vi "StDev Filter Demonstrator.vi"() -> ()   [LabVIEW 2011]
uses:
  <vilib>/ptbypt/NI_PtbyPt.lvlib
  <vilib>/Utility/file.llb/Read From Spreadsheet File (DBL).vi
panel:
  out "Numeric":i32
  out "element":dbl
  in  "shot":dbl=0.8 step=0.01
  out "Waveform Chart":cluster{dbl, dbl}(graph)
  in  "sample":i32=3
  out "Filtered Value":dbl
  in  "StDev":dbl=0.05 step=0.001
  out "StDev":dbl format="%0.2f"
  out "I+N":dbl
  in  "Input":dbl step=0.1
  in  "Manual":bool
  in  "noise":dbl(knob)=0.05940857995844632 scale=0.0..0.1
  in  "Use Time ?":bool=TRUE
  in  "frequency":dbl=0.0001 format="%0.4e"
  in  "amplitude":dbl=0.9999999999999999 step=0.1 format="%0.2f"
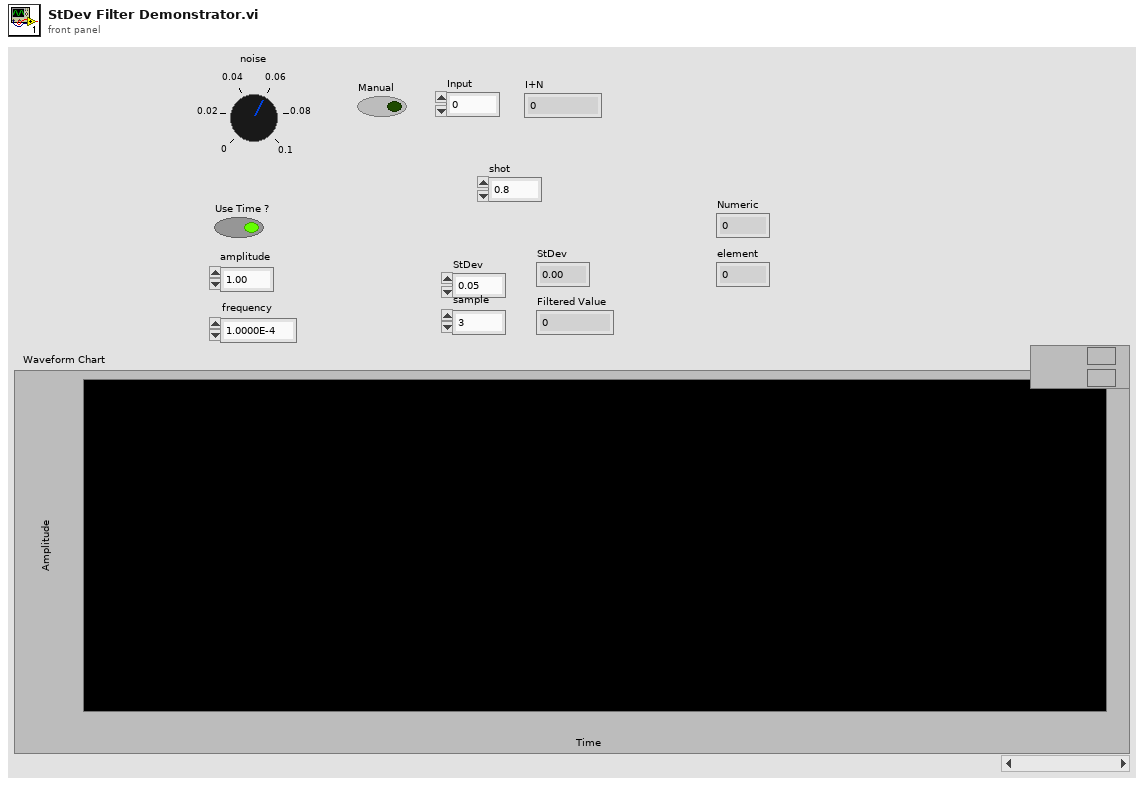
[diagram p1: front panel]
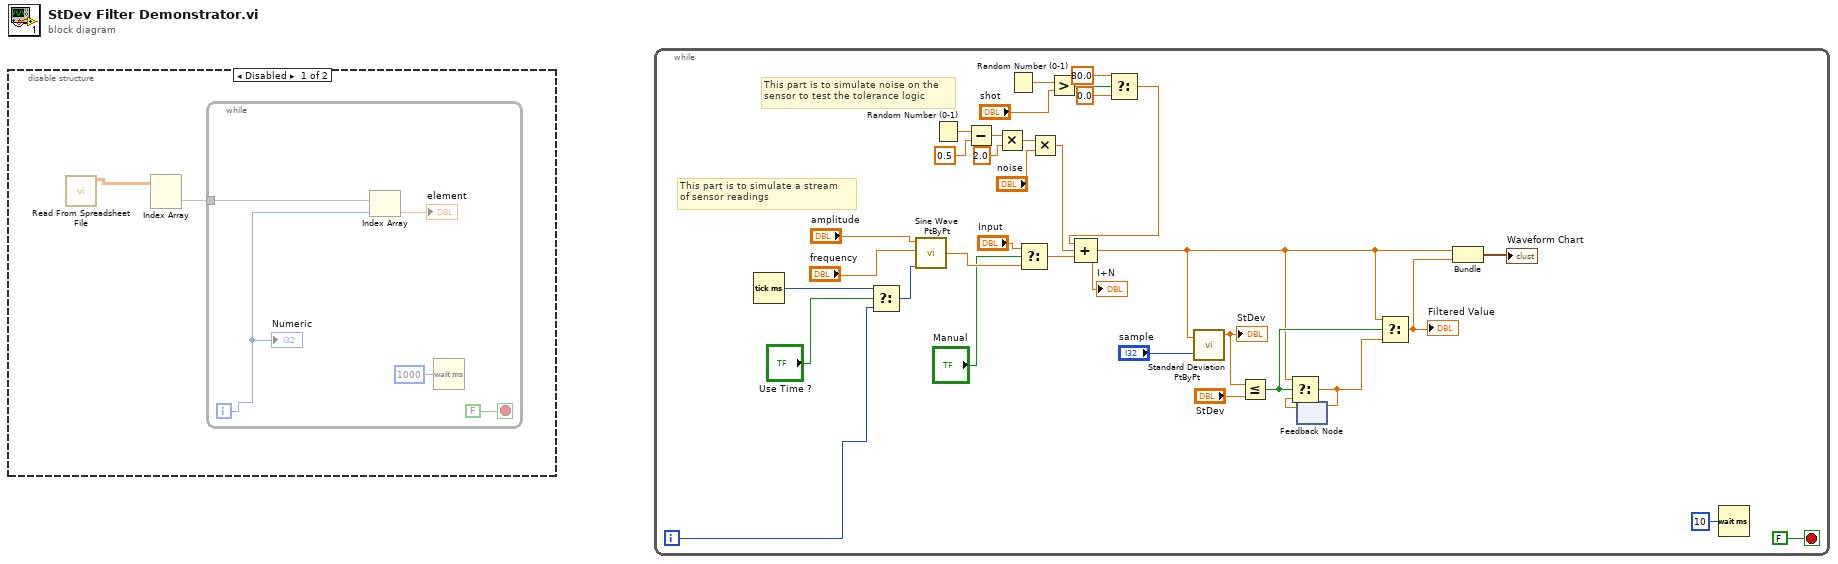
[diagram p0: block diagram]
diagram:
  n1 = disable-structure shown="Disabled" {
    frame Disabled {
      n2 = call-poly <vilib>:"Read From Spreadsheet File.vi"() -> ("all rows"=w2:dbl[][])  [unwired: 7 in, 4 out]
      n3 = Index Array(array=w2) -> (element=w1:dbl[])  [unwired: 2 in]
      n4 = while {
        tunnel: w1 -> [w6]
        i -> [w7]
        stop <- FALSE stop-if-true
        n5 = Index Array(array=w6, index=w7) -> (element=→"element":dbl)
        n6 = Wait (ms)(milliseconds to wait=u32 1000) -> ()  [unwired: 1 out]
        "Numeric" <- w7
      }
    }
    frame Enabled {
    }
  }
  n7 = while {
    i -> [w11]
    stop <- FALSE stop-if-true
    # "This part is to simulate noise on the \nsensor to test the tolerance logic"
    # "This part is to simulate a stream\nof sensor readings"
    n8 = Tick Count (ms)() -> (millisecond timer value=w10:u32)
    n9 = Select(t=w10, s="Use Time ?", f=w11) -> (s? t:f=w27:u32)
    n10 = call <vilib>:"Sine Wave PtByPt.vi"("time"=w27, "frequency"="frequency", "amplitude"="amplitude") -> ("sine wave"=w38:dbl)  [unwired: 1 in]
    n11 = Random Number (0-1)() -> (number: 0 to 1=w29:dbl)
    n12 = Subtract(x=w29, y=0.5) -> (x-y=w31:dbl)
    n13 = Multiply(x=w31, y=2.0) -> (x*y=w33:dbl)
    n14 = Random Number (0-1)() -> (number: 0 to 1=w17:dbl)
    n15 = Select(t="Input", s="Manual", f=w38) -> (s? t:f=w36:dbl)
    n16 = Multiply(x=w33, y="noise") -> (x*y=w35:dbl)
    n17 = Greater?(x=w17, y="shot") -> (0:w14:bool)
    n18 = Select(t=80.0, s=w14, f=0.0) -> (s? t:f=w15:dbl)
    n19 = Compound Arithmetic op=ADD(w15, w35, w36) -> (w9:dbl)
    "I+N" <- w9
    n20 = call <vilib>:"Standard Deviation PtByPt.vi"("x"=w9, "sample length"="sample") -> ("standard deviation"=w24:dbl)  [unwired: 1 in, 2 out]
    "StDev" <- w24
    n21 = Less Or Equal?(x=w24, y="StDev") -> (x <= y?=w21:bool)
    n22 = feedback #1() -> (w22:dbl)  [unwired: 1 in]
    n23 = Select(t=w9, s=w21, f=w22) -> (s? t:f=w8:dbl)
    n24 = feedback-in #1(w8) -> ()
    n25 = Select(t=w9, s=w21, f=w8) -> (s? t:f=w19:dbl)
    "Filtered Value" <- w19
    n26 = Bundle(w9, w19) -> (→"Waveform Chart":cluster{dbl, dbl})  [unwired: 1 in]
    n27 = Wait (ms)(milliseconds to wait=u32 10) -> ()  [unwired: 1 out]
  }
